vi "Write active scale index .vi"(8 "error in (no error)":errorcluster, 10 "active scale index":i32, 11 "Scaling editor node in":refnum<class "Scaling editor node.lvclass">) -> (0 "error out":errorcluster, 3 "Scaling editor node out":refnum<class "Scaling editor node.lvclass">)   [LabVIEW 2013, in "Scaling editor node.lvclass"]
uses:
  Scaling editor node.lvclass
  Scaling editor node.lvclass/Scaling editor node.ctl
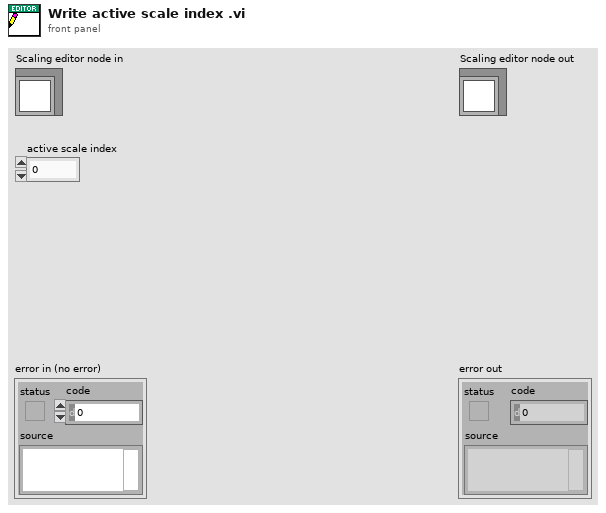
[diagram p1: front panel]
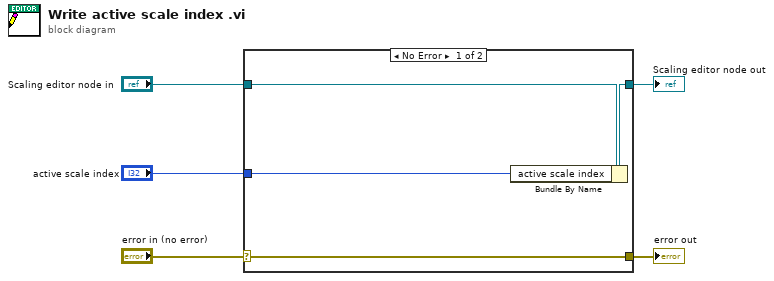
[diagram p0: block diagram]
diagram:
  n1 = case shown="No Error" "error in (no error)" {
    selector: "error in (no error)" -> [w9 w10]
    tunnel: [w9 w10] -> w4
    tunnel: [w7 w11] -> w2
    tunnel: "Scaling editor node in" -> [w8 w11]
    tunnel: "active scale index" -> [w6 _]
    frame No Error {
      n2 = Bundle By Name(cluster=w8, "active scale index"=w6) -> (w7:refnum<class "Scaling editor node.lvclass">)
    }
    frame Error {
    }
  }
  "error out" <- w4
  "Scaling editor node out" <- w2
